vi "DSD-VA_carac_y=aX-n0@4.vi"(8 "error in (no error)":errorcluster caption="err in", 9 "S_X":dbl, 10 "E(X)":dbl, 11 "a":dbl) -> (0 "error out":errorcluster caption="err out", 1 "S_aX":dbl, 2 "E(a.X)":dbl)   [LabVIEW 2010, in "lv_02.lvlib"]
doc: "Soit une variable X de moyenne E(X) et d'écart-type S_X alors si Y est une variable telle que Y=a.X, alors on a E(Y)=E(aX)=a.E(X) et S_Y=S_aX=Racine(a)*S_aX\nCas particulier : si l'écart-type S_X n'est pas donné (=0) et que E(X) est faible, selon le modèle de Poisson, on a S_aY=Racine[E(Y)]"
uses:
  lv_02.lvlib
panel:
  # "Soit une variable X de moyenne E(X) et d'écart-type S_X alors si Y est une variable telle que Y=a.X, alors on a E(Y)=E(aX)=a.E(X) et S_Y=S_aX=Racine(a)*S_aX\nCas particulier : si l'écart-type S_X n'est pas donné (=0) et que E(X) est faible, selon le modèle de Poisson, on a S_aY=Racine[E(Y)]"
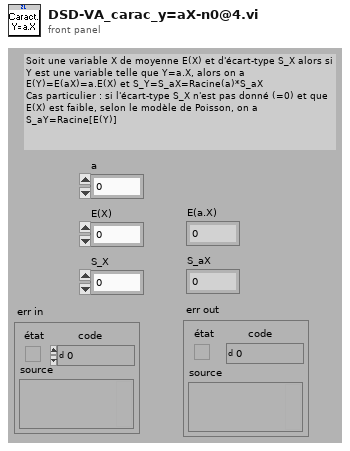
[diagram p1: front panel]
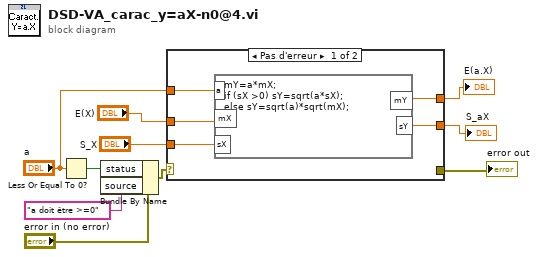
[diagram p0: block diagram]
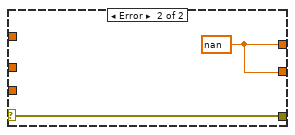
[diagram p2: hidden frame]
diagram:
  n1 = Less Or Equal To 0?(x="a") -> (x <= 0?=w9:bool)
  n2 = Bundle By Name(cluster="error in (no error)", "status"=w9, "source"="a doit être >=0") -> (w7:errorcluster)
  n3 = case shown="Pas d'erreur" w7 {
    selector: w7 -> [_ w16]
    tunnel: [_ w16] -> w10
    tunnel: "a" -> [w15 _]
    tunnel: "E(X)" -> [w14 _]
    tunnel: "S_X" -> [w13 _]
    tunnel: [w12 w17] -> w3
    tunnel: [w11 w17] -> w2
    frame No Error {
      n4 = formula code="mY=a*mX;\nif (sX >0) sY=sqrt(a*sX);\nelse sY=sqrt(a)*sqrt(mX);"("a"=w15, "mX"=w14, "sX"=w13) -> ("mY"=w12:dbl, "sY"=w11:dbl)
    }
    frame Error {
      w17 = nan ("mY")
    }
  }
  "error out" <- w10
  "E(a.X)" <- w3
  "S_aX" <- w2
